vi "cnvrt_waveNr_nmAir.vi"(0 "reference in":refnum<class "OSA.lvclass">, 2 "waveNr":dbl format="%.2f", 5 "error in (no error)":errorcluster) -> (14 "reference out":refnum<class "OSA.lvclass">, 16 "wavelength (nmAir)":dbl format="%.2f", 19 "error out":errorcluster)   [LabVIEW 2010, in "OSA.lvclass"]
doc: "Note! this vi requires prior reading of all environment parameters, \n(temperature, pressure and humidity).\n\nUse the environment_get.vi!"
uses:
  OSA.lvclass
  FTSLib.dll
panel:
  # "Note! this vi requires prior reading of all environment parameters, \n(temperature, pressure and humidity).\n\nUse the environment_get.vi!"
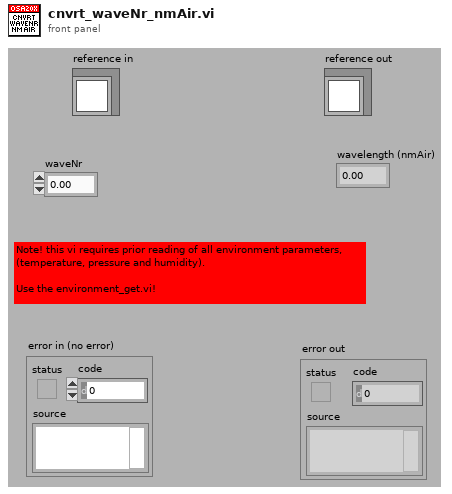
[diagram p1: front panel]
types:
  T1 = typedef "OSA.lvclass/ObjectAttributes.ctl" = cluster{"Stop":bool, "dataType":T2, "spectrometerIdx":u16, "buffer size interferogram":i32, "interferogram":cluster{"new":bool, "plot_x_ min":sgl, "plot_x_max":sgl, "plot_y_min":sgl, "plot_y_max":sgl, "Graph Intrfrgrm":T3, "timeStamp":u32, "signal (%)":dbl, "traces":cluster{"idx":u32, "broadBand":bool, "monoChromatic":bool, "peakToPeakSignal":dbl, "peakToPeakPos":dbl}[], "traces idx last":i32}, "spectrum":cluster{"new":bool, "plot_x_min":sgl, "plot_x_max":sgl, "plot_unit_x":T4, "plot_unit_y":T5, "plot_y_min":sgl, "plot_y_max":sgl, "Graph Spectrum":T3, "timeStamp":u32, "X_VAL_OPTIONS":enum16{"MIN_MAX", "ARRAY"}, "traces":cluster{"idx":u32}[], "traces idx last":i32}, "Thorlabs_OSA_64.lvclass:queue_action.ctlqueue ref":refnum<queue>, "action":T6, "plot zoom step":dbl, "buffer semaphore":T7, "acq stopped":bool, "dataType active":T2, "temperature (degr C)":sgl, "pressure (hPa)":sgl, "rel humidity (%)":sgl, "settings":cluster{"resolution":T8, "sensitivity":T9, "Average":bool, "average nr":u32, "apodisation":T10, "acq delay (ms)":u32, "airMesure":T11, "wmtr on":bool, "intfgrm_smooth_width":u16, "intfgrm_smooth_nrOfPasses":u16, "intfgrm_smooth":T12, "phaseCorrection":T13, "zeroFill":u8, "spectr_smooth":T12, "spectr_smooth_width":u16, "spectr_smooth_nrOfPasses":u16, "resolution (/cm)":sgl, "REF wavelength, (nm)":dbl, "gain_idx":u16, "gainAuto":bool, "gain_relative":dbl, "PD sensitivity mode":T14, "PD senseMode implemented":bool, "SensorTemperature implemented":bool, "SensorPressure implemented":bool, "SensorHumidity implemented":bool}, "peaks position":sgl[], "peaks width":sgl[], "peaks height":sgl[], "peaks max nr":u32, "peaks latest nr":i32, "peaks new":bool, "power":dbl, "power new":bool, "path":string, "wavelength (WNr)":dbl, "wavelength new":bool, "buffer size spectrum":i32, "status":string, "VI reference":refnum<vi>, "funcPointer":u64, "libraryPointer":u64, "singleAcquisition":bool, "coherenceLength (cm)":dbl, "coherenceLength new":bool, "spectrometer model":string, "spectrometer serial nr":string, "peaks thld left":sgl[], "peaks thld right":sgl[], "coherenceLength error (cm)":dbl, "ADC bits":u16, "peaks position centroid":sgl[], "peaks height centroid":sgl[], "OSA series":T15, "channel":u16, "channels_nr":i32, "channel stiched":u32}
  T2 = typedef "OSA.lvclass/acq_dataType.ctl" = enum16{"none", "interferogram", "spectrum"}
  T3 = typedef "OSA.lvclass/graph_intensity.ctl" = refnum<vi>
  T4 = typedef "OSA.lvclass/spectrum_x_unit.ctl" = enum16{"wavenr/cm", "THz", "eV", "nm_air", "nm_vac"}
  T5 = typedef "OSA.lvclass/y_unit.ctl" = enum16{"ADC counts", "dBm pwr absolute", "dBm pwr density", "mW pwr absolute", "mW pwr density"}
  T6 = typedef "OSA.lvclass/queue_action.ctl" = enum16{"none", "stop", "GUI_plotInterferogram", "GUI_plotSpectrum", "GUI_plotInterferogramRescale", "GUI_plotSpectrumRescale", "GUI_plotInterferogramReset", "GUI_plotSpectrumReset", "GUI_plotInterferogramAutoScaleY", "GUI_plotSpectrumAutoScaleY", "GUI_plotInterferogramZoomOut", "GUI_plotSpectrumZoomOut", "GUI_plotInterferogramPane", "GUI_plotSpectrumPane", "GUI_plotInterferogramZoomMouse", "GUI_plotSpectrumZoomMouse", "ENVIRONMENT temperature", "ENVIRONMENT pressure", "MODE_resolution set", "MODE_resolution get", "MODE_sensitivity set", "MODE_sensitivity get", "MODE_PDTemperature set", "MODE_PDTemperature get", "REBOOT/RESET firmware", "ACQASYNC_acquireSingleSpectrum", "ACQASYNC_continuous start", "ACQASYNC_continuous stop\n", "ACQASYNC_get last interferogram", "ACQASYNC_get last spectrum", "ACQASYNC_get last waveNr", "ACQOPT_interferogram smoothing set", "ACQOPT_interferogram smoothing get", "ACQOPT_spectrum smoothing set", "ACQOPT_spectrum smoothing get", "ACQOPT_apodisation type set", "ACQOPT_apodisation type get", "ACQOPT_phase correction type set", "ACQOPT_phase correction type get", "ACQOPT_acqIntervall_set", "ACQOPT_acqIntervall_get", "ACQOPT_average spectrum set", "ACQOPT_average spectrum get", "ACQOPT_rolling average set", "ACQOPT_rolling average get", "ACQOPT_zero fill factor set", "ACQOPT_zero fill factor get", "ACQOPT_cycle counting set", "ACQOPT_cycle counting get", "ACQOPT_air measure option set", "ACQOPT_air measure option get", "ACQOPT_gainLevel auto get", "ACQOPT_gainLevel auto set", "ACQOPT_gainLevel get", "ACQOPT_gainLevel set", "ACQOPT_getAll", "INSTRUMENT_PROPERTY_range_WaveNr_min", "INSTRUMENT_PROPERTY_range_WaveNr_max", "INSTRUMENT_PROPERTY_reference_wavelength_cm^-1", "INSTRUMENT_PROPERTY_samplesPerRefPeriod", "INSTRUMENT_PROPERTY_resolution_waveNrPercm", "INSTRUMENT_PROPERTY_availableGainLevels", "INSTRUMENT_PROPERTY_status", "CONVERT", "ANALYSE_POWER", "ANALYSE_PEAKS", "ANALYSE_WAVELENGTH", "ANALYSE_SPECTRUM", "ANALYSE_INTERFEROGRAM", "ANALYSE_COHERENCE_LENGTH", "MATH", "MATH_power", "MATH_peaks", "FILE", "miscellaneous"}
  T7 = typedef "Semaphore RefNum" = refnum<k1>
  T8 = typedef "OSA.lvclass/resolution.ctl" = enum16{"low", "high"}
  T9 = typedef "OSA.lvclass/sensitivityMode.ctl" = enum16{"low", "low medium", "high medium", "high"}
  T10 = typedef "OSA.lvclass/apodisation.ctl" = enum16{"NONE", "NORTON_BEER_WEAK", "NORTON_BEER_MEDIUM", "NORTON_BEER_STRONG", "TRIANGULAR", "COSINE", "HANN", "HAMMING", "BLACKMANHARRIS3", "BLACKMANHARRIS4", "GAUSSIAN"}
  T11 = typedef "OSA.lvclass/airMeasure.ctl" = enum16{"TEMPERATURE", "PRESSURE"}
  T12 = typedef "OSA.lvclass/smoothing.ctl" = enum16{"NONE", "BINOMIAL", "SAVITSKY_GOLAY", "FOURIER", "MOVING_AVERAGE", "GAUSSIAN"}
  T13 = typedef "OSA.lvclass/phaseCorrection.ctl" = enum16{"NONE", "MERTZ", "FORMAN", "MERTZ_FILE", "FORMAN_FILE", "FUTURE COMP."}
  T14 = typedef "OSA.lvclass/PDTemperatureMode.ctl" = enum16{"cool: better sensitivity/noise floor", "warm: extended wl range"}
  T15 = typedef "OSA_series.ctl" = enum16{"OSA200", "OSA300", "UNKNOWN"}
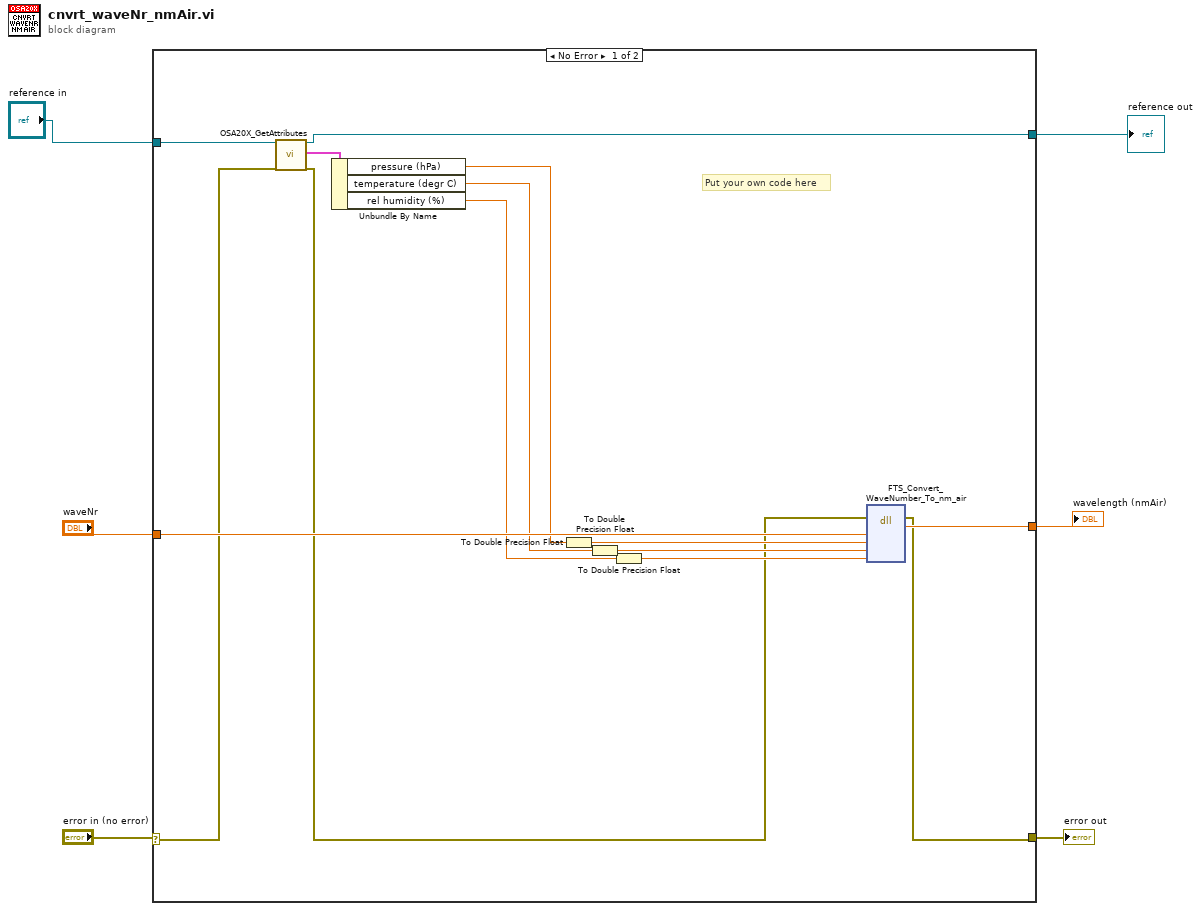
[diagram p0: block diagram]
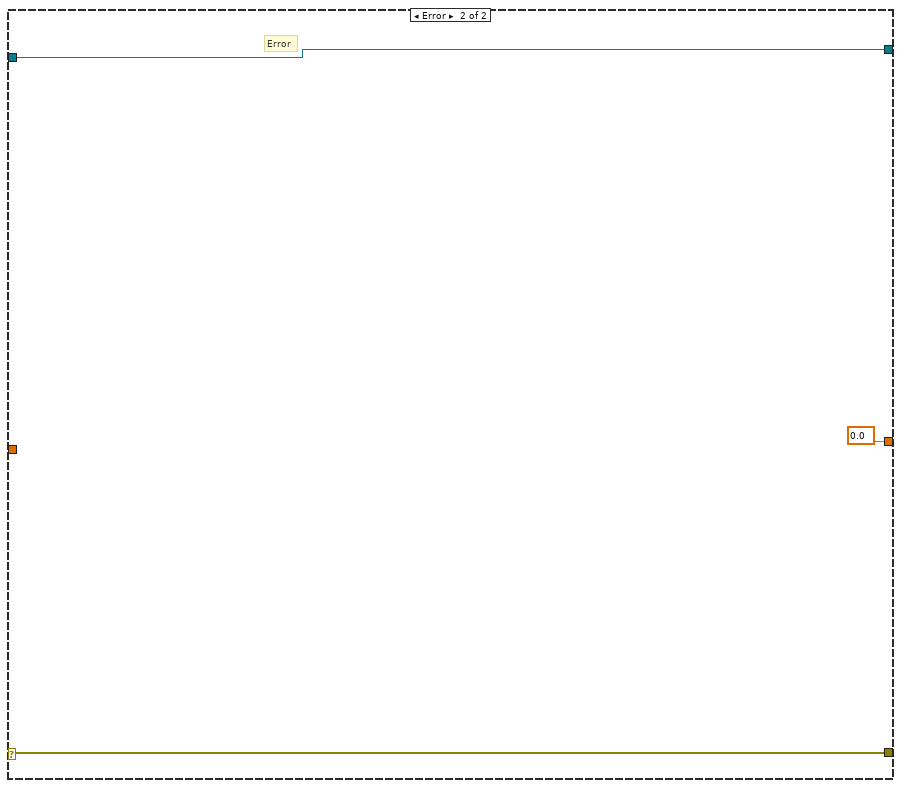
[diagram p2: hidden frame]
diagram:
  n1 = case shown="No Error" "error in (no error)" {
    selector: "error in (no error)" -> [w11 w23]
    tunnel: [w9 w23] -> w6
    tunnel: "waveNr" -> [w20 _]
    tunnel: [w19 0.0] -> w3
    tunnel: "reference in" -> [w8 w21]
    tunnel: [w7 w21] -> w1
    frame No Error {
      # "Put your own code here"
      n2 = call "OSA20X_GetAttributes.vi"("reference in"=w8, "error in (no error)"=w11) -> ("reference out"=w7:refnum<class "OSA.lvclass">, "Data"=w18:T1, "error out"=w10:errorcluster)  [unwired: 14 in, 1 out]
      n3 = Unbundle By Name(w18) -> ("pressure (hPa)"=w17:sgl, "temperature (degr C)"=w16:sgl, "rel humidity (%)"=w15:sgl)
      n4 = To Double Precision Float(number=w17) -> (double precision float=w14:dbl)
      n5 = To Double Precision Float(number=w16) -> (double precision float=w13:dbl)
      n6 = To Double Precision Float(number=w15) -> (double precision float=w12:dbl)
      n7 = dll-call lib="FTSLib.dll" fn="FTS_Convert_WaveNumber_To_nm_air"(error in=w10, "waveNr"=w20, "pressure"=w14, "airTemp"=w13, "relHumidity"=w12) -> (error out=w9:errorcluster, "return type"=w19:dbl)  [unwired: 6 in, 1 out]
    }
    frame Error {
      # "Error"
    }
  }
  "error out" <- w6
  "wavelength (nmAir)" <- w3
  "reference out" <- w1
